vi "Dashboard Main.vi"() -> ()   [LabVIEW 2017]
uses:
  <vilib>/Utility/miscctls.llb/LVRowAndColumnTypeDef.ctl
  <vilib>/event_ctls.llb/eventvkey.ctl
  <vilib>/Rock Robotics/Network Tables/NT Read Numeric Array.vi
  <vilib>/Rock Robotics/WPI/Dashboard/WPI_DashboardLogging Global.vi
panel:
  in  "Camera Settings Right":T1={"Frame Rate"=30, "Compression"=30, "Size"=1, "DB Camera Config"=FALSE} {"Frame Rate" scale=1.0..30.0; "Compression" scale=100.0..-1.0; "Size" items=["640x480", "320x240", "160x120"]}
  in  "Camera Name Right":string(combo)="No Camera Selection"
  out "Camera Info":cluster{"Mbps LED":bool, "Mbps":dbl, "fps":dbl} {"fps" format="%#.1g"; "Mbps" format="%#.1g"}
  in  "Camera Settings":T1={"Frame Rate"=30, "Compression"=30, "Size"=1, "DB Camera Config"=FALSE} {"Frame Rate" scale=1.0..30.0; "Compression" scale=100.0..-1.0; "Size" items=["640x480", "320x240", "160x120"]}
  in  "TCP":refnum<k5>
  in  "Rec Mode":enum32{"Stop", "Record", "Playback"}(radio)
  out "Robot IP":string
  out "Image Message":string="Timeout in Camera Communications"
  in  "Dashboard Tab":T2(tab)
  in  "Select Robot Start Location":string(combo)="Select Robot Start Position ..."
  in  "String":string="Tom's Custom Dashboard 2018"
  in  "Select Auto":string(combo)="Select Autonomous ..."
  out "NT Connection":bool
  out "MotorChart R":cluster{"Numeric":dbl, "Numeric":dbl}(graph)
  out "MotorChart L":cluster{"Numeric":dbl, "Numeric":dbl}(graph)
  out "MotorSliders R":cluster{"MotorSlide1":dbl, "MotorSlide2":dbl} {"MotorSlide2" scale=-1.0..1.0 scale format="%#_2e"; "MotorSlide1" scale=-1.0..1.0 scale format="%#_2e"}
  out "MotorSliders L":cluster{"MotorSlide1":dbl, "MotorSlide2":dbl} {"MotorSlide2" scale=-1.0..1.0 scale format="%#_2e"; "MotorSlide1" scale=-1.0..1.0 scale format="%#_2e"}
  out "Gyro":dbl(knob) scale=0.0..360.0
  out "JS1 Z":dbl(slide) scale=-1.0..1.0 scale format="%#_2e"
  out "JS1 Graph":cluster{"X":dbl, "Y":dbl}[](graph)
  out "JS1 Buttons":T3
  out "JS2 Z":dbl(slide) scale=-1.0..1.0 scale format="%#_2e"
  out "JS2 Graph":cluster{"X":dbl, "Y":dbl}[](graph)
  out "JS2 Buttons":T3
  out "Mode":T4(ring)=enum."Auto Disabled"
  out "Camera Image Right":T5(plugin-control)
  in  "DB/String 9":string
  in  "DB/String 8":string
  in  "DB/String 7":string
  in  "DB/String 6":string
  in  "DB/String 5":string
  in  "DB/String 4":string
  in  "DB/String 3":string
  in  "DB/String 2":string
  in  "DB/String 1":string
  in  "DB/String 0":string
  in  "DB/Slider 0":dbl(slide) scale=0.0..5.0
  in  "DB/Slider 1":dbl(slide) scale=0.0..5.0
  in  "DB/Slider 2":dbl(slide) scale=0.0..5.0
  in  "DB/Slider 3":dbl(slide) scale=0.0..5.0
  out "DB/LED 3":bool
  out "DB/LED 2":bool
  out "DB/LED 1":bool
  out "DB/LED 0":bool
  in  "DB/Button 3":bool
  in  "DB/Button 2":bool
  in  "DB/Button 1":bool
  in  "DB/Button 0":bool caption="New Name"
  in  "Test Slider":dbl(slide) scale=0.0..100.0 scale format="%#_3g"
  in  "On/Off":bool caption="Solenoid"
  in  "Test Name":u16(ring) items=["Select the test to run..."]
  in  "Test Tree":string(tree)
  in  "Motor":cluster{"Value":dbl, "Enable":bool} {"Value" scale=-1.0..1.0 scale format="%#_3g"}
  out "Progress":T6 {"Test Progress" scale=0.0..100.0}
  in  "Rev/Fwd":cluster{"Forward":bool, "Reverse":bool}
  in  "Test Ring":u16(ring) items=["Monochrome", "Color"]
  out "Cmd Status":string
  in  "Execute Command":bool
  in  "Command Params":string[][](table)
  in  "Command Selection":i32(listbox)
  in  "CheckList":i32(listbox)
  out "Tree":string(tree)
  out "Camera Image":T5(plugin-control)
  out "Background":bool
  in  "Camera Name":string(combo)="No Camera Selection"
  # "HW"
  # "HW"
  # "Joysticks"
  # "Drive Motors"
  # "Front"
  # "Right"
  # "Left"
  # "Back"
  # "This tab is a great place for autonomous settings and robot-specific values.\nPlace controls and indicators inside this tab and match name to\nDashboard Variables on robot. You can also delete this comment."
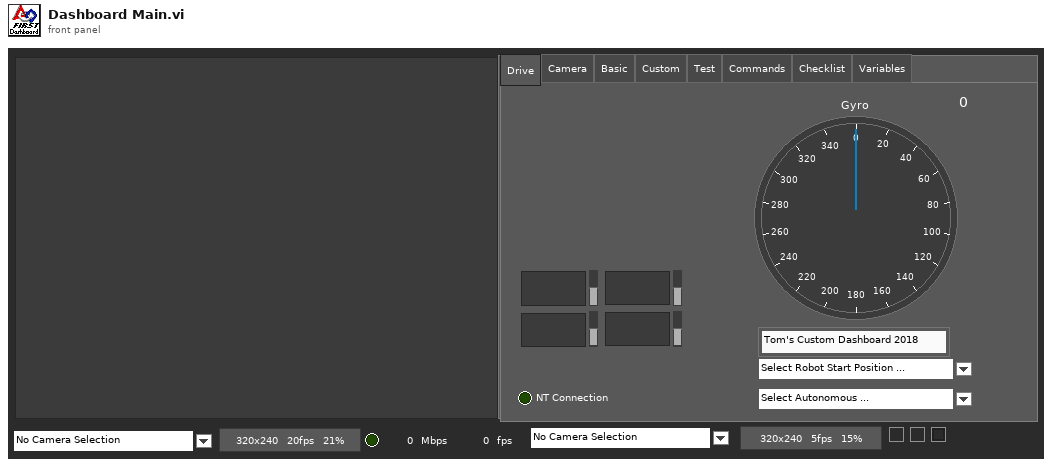
[diagram p1: front panel]
types:
  T1 = cluster{"Frame Rate":i32, "Compression":i32, "Size":u16, "DB Camera Config":bool}
  T2 = enum32{"Drive", "Camera", "Basic", "Custom", "Test", "Commands", "Checklist", "Variables"}
  T3 = cluster{bool, bool, bool, bool, bool, bool, bool, bool, bool, bool, bool, bool}
  T4 = enum8{"Tele-Op Disabled", "Tele-Op Enabled", "Auto Disabled", "Auto Enabled", "Test Disabled", "Test Enabled", "Disconnected", "No Code", "E-Stop"}
  T5 = typedef "IMAQ Image.ctl" = refnum<image>
  T6 = cluster{"Test Progress":u8, "Test Progress Text":string}
  T7 = cluster{"Save Path":path, "Interval (s)":dbl, "Keep":i32}
  T8 = typedef "Image Type" = u32
  T9 = cluster{"IDs":cluster{"RPC field ID":u16, "Unique ID":u16}, "String":string}
  T10 = cluster{"Error Strings":string, "Disable Counts":cluster{u16, u16}, "Rail Faults":cluster{u16, u16, u16}, "Robot IP":string, "DB Mode":u8, "Event Info":cluster{"Name":string, "Type":u8, "Number":u16, "Replay":u8}}
  T11 = cluster{"Storage":cluster{"Disk Free":u64, "RAM Block":u32, "RAM free":u32}, "CPU Utilization":cluster{"CPU % ISR":sgl, "CPU % Time Crit":sgl, "CPU % Timed Str":sgl, "CPU % High":sgl, "CPU % Above":sgl, "CPU % Normal":sgl, "CPU % Low":sgl}, "CAN":cluster{"% Bus Utilization":sgl, "Bus Off Cnt":u32, "TX_FIFO Full Cnt":u32, "Receive Error Cnt":u8, "Transmit Error Cnt":u8}, "HID":cluster{"HID Outputs":u32, "Rumble Low":u16, "Rumble High":u16}[]}
  T12 = cluster{"Status bits":cluster{"Test Mode":bool, "Autonomous":bool, "Enabled":bool, "Code Start":bool, "Brownout":bool, "Reserved 2":bool, "Reserved 3":bool, "E-Stop":bool}, "Code Trace":cluster{"Disabled":bool, "TeleOp":bool, "Auto":bool, "Test":bool}, "Controller Type":enum16{"unknown", "cRIO", "roboRio"}, "Code?":enum16{"unknown", "noCode", "code"}, "Battery V":dbl}
  T13 = cluster{"Control Bits":cluster{"TestMode":bool, "Autonomous":bool, "Enabled":bool, "FMS Present":bool, bool, bool, bool, "E-Stop":bool}, "Team Station ":u8, "Countdown":sgl, "Joystick Values":cluster{"Axes":dbl[], "Buttons":bool[], "POVs":i16[]}[]}
  T14 = cluster{"Axes":dbl[], "Buttons":bool[], "POVs":i16[]}[]
  T15 = cluster{"Axes":dbl[], "Buttons":bool[], "POVs":i16[]}
  T16 = cluster{"Buttons[0]":bool, "Buttons[1]":bool, "Buttons[2]":bool, "Buttons[3]":bool, "Buttons[4]":bool, "Buttons[5]":bool, "Buttons[6]":bool, "Buttons[7]":bool, "Buttons[8]":bool, "Buttons[9]":bool, "Buttons[10]":bool, "Buttons[11]":bool}
  T17 = cluster{"Camera Image":refnum<vi>, "Dashboard Tab":refnum<vi>, "Background":refnum<vi>, "Rec Mode":refnum<vi>, "Test Slider":refnum<vi>, "On/Off ":refnum<vi>, "Test Ring":refnum<vi>, "Rev/Fwd":refnum<vi>, "Test Name":refnum<vi>, "Motor":refnum<vi>, "Progress":refnum<vi>, "CheckList":refnum<vi>, "Tree":refnum<vi>, "Test Tree":refnum<vi>, "Command Params":refnum<vi>, "Command Selection":refnum<vi>, "Execute Command":refnum<vi>, "Cmd Status":refnum<vi>, "Camera Settings":refnum<vi>, "Camera Name":refnum<vi>, "Camera Info":refnum<vi>, "Camera Settings Right":refnum<vi>, "Camera Name Right":refnum<vi>, "Camera Image Right":refnum<vi>}
  T18 = cluster{"Camera Name":string, string, "Saved DB Images Info":cluster{"Save Path":path, "Interval (s)":dbl, "Keep":i32}}
  T19 = cluster{"Camera Name Right":string, string, "Saved DB Images Info":cluster{"Save Path":path, "Interval (s)":dbl, "Keep":i32}}
  T20 = cluster{"Operation":enum16{"Update", "Clear"}, "Color Box":u32}[]
  T21 = typedef "eventvkey.ctl" = enum16{"ASCII", "Enter", "Return", "Shift", "Ctrl", "Alt", "Cmd", "Opt", "Caps", "NumLock", "Clear", "Break", "Up", "Down", "Left", "Right", "Insert", "Delete", "Home", "End", "PageUp", "PageDown", "Escape", "Help", "Pause", "ScrollLock", "F1", "F2", "F3", "F4", "F5", "F6", "F7", "F8", "F9", "F10", "F11", "F12", "F13", "F14", "F15", "F16", "F17", "F18", "F19", "F20", "F21", "F22", "F23", "F24", "Play", "VolumeUp", "VolumeDown", "Mute", "Two Byte Char"}
  T22 = cluster{"Image Size":bool, "Image Type":bool, "Pixel Value":bool, "ROI Information":bool, "Zoom Factor":bool}
  T23 = cluster{"Operation":enum16{"Update", "Clear"}, "Color Box":u32}
  T24 = typedef "LVRowAndColumnTypeDef.ctl" = cluster{"Row":i32, "Column":i32}
  T25 = cluster{"Shift":bool, "Ctrl":bool, "Alt":bool, "Cmd":bool, "Opt":bool}
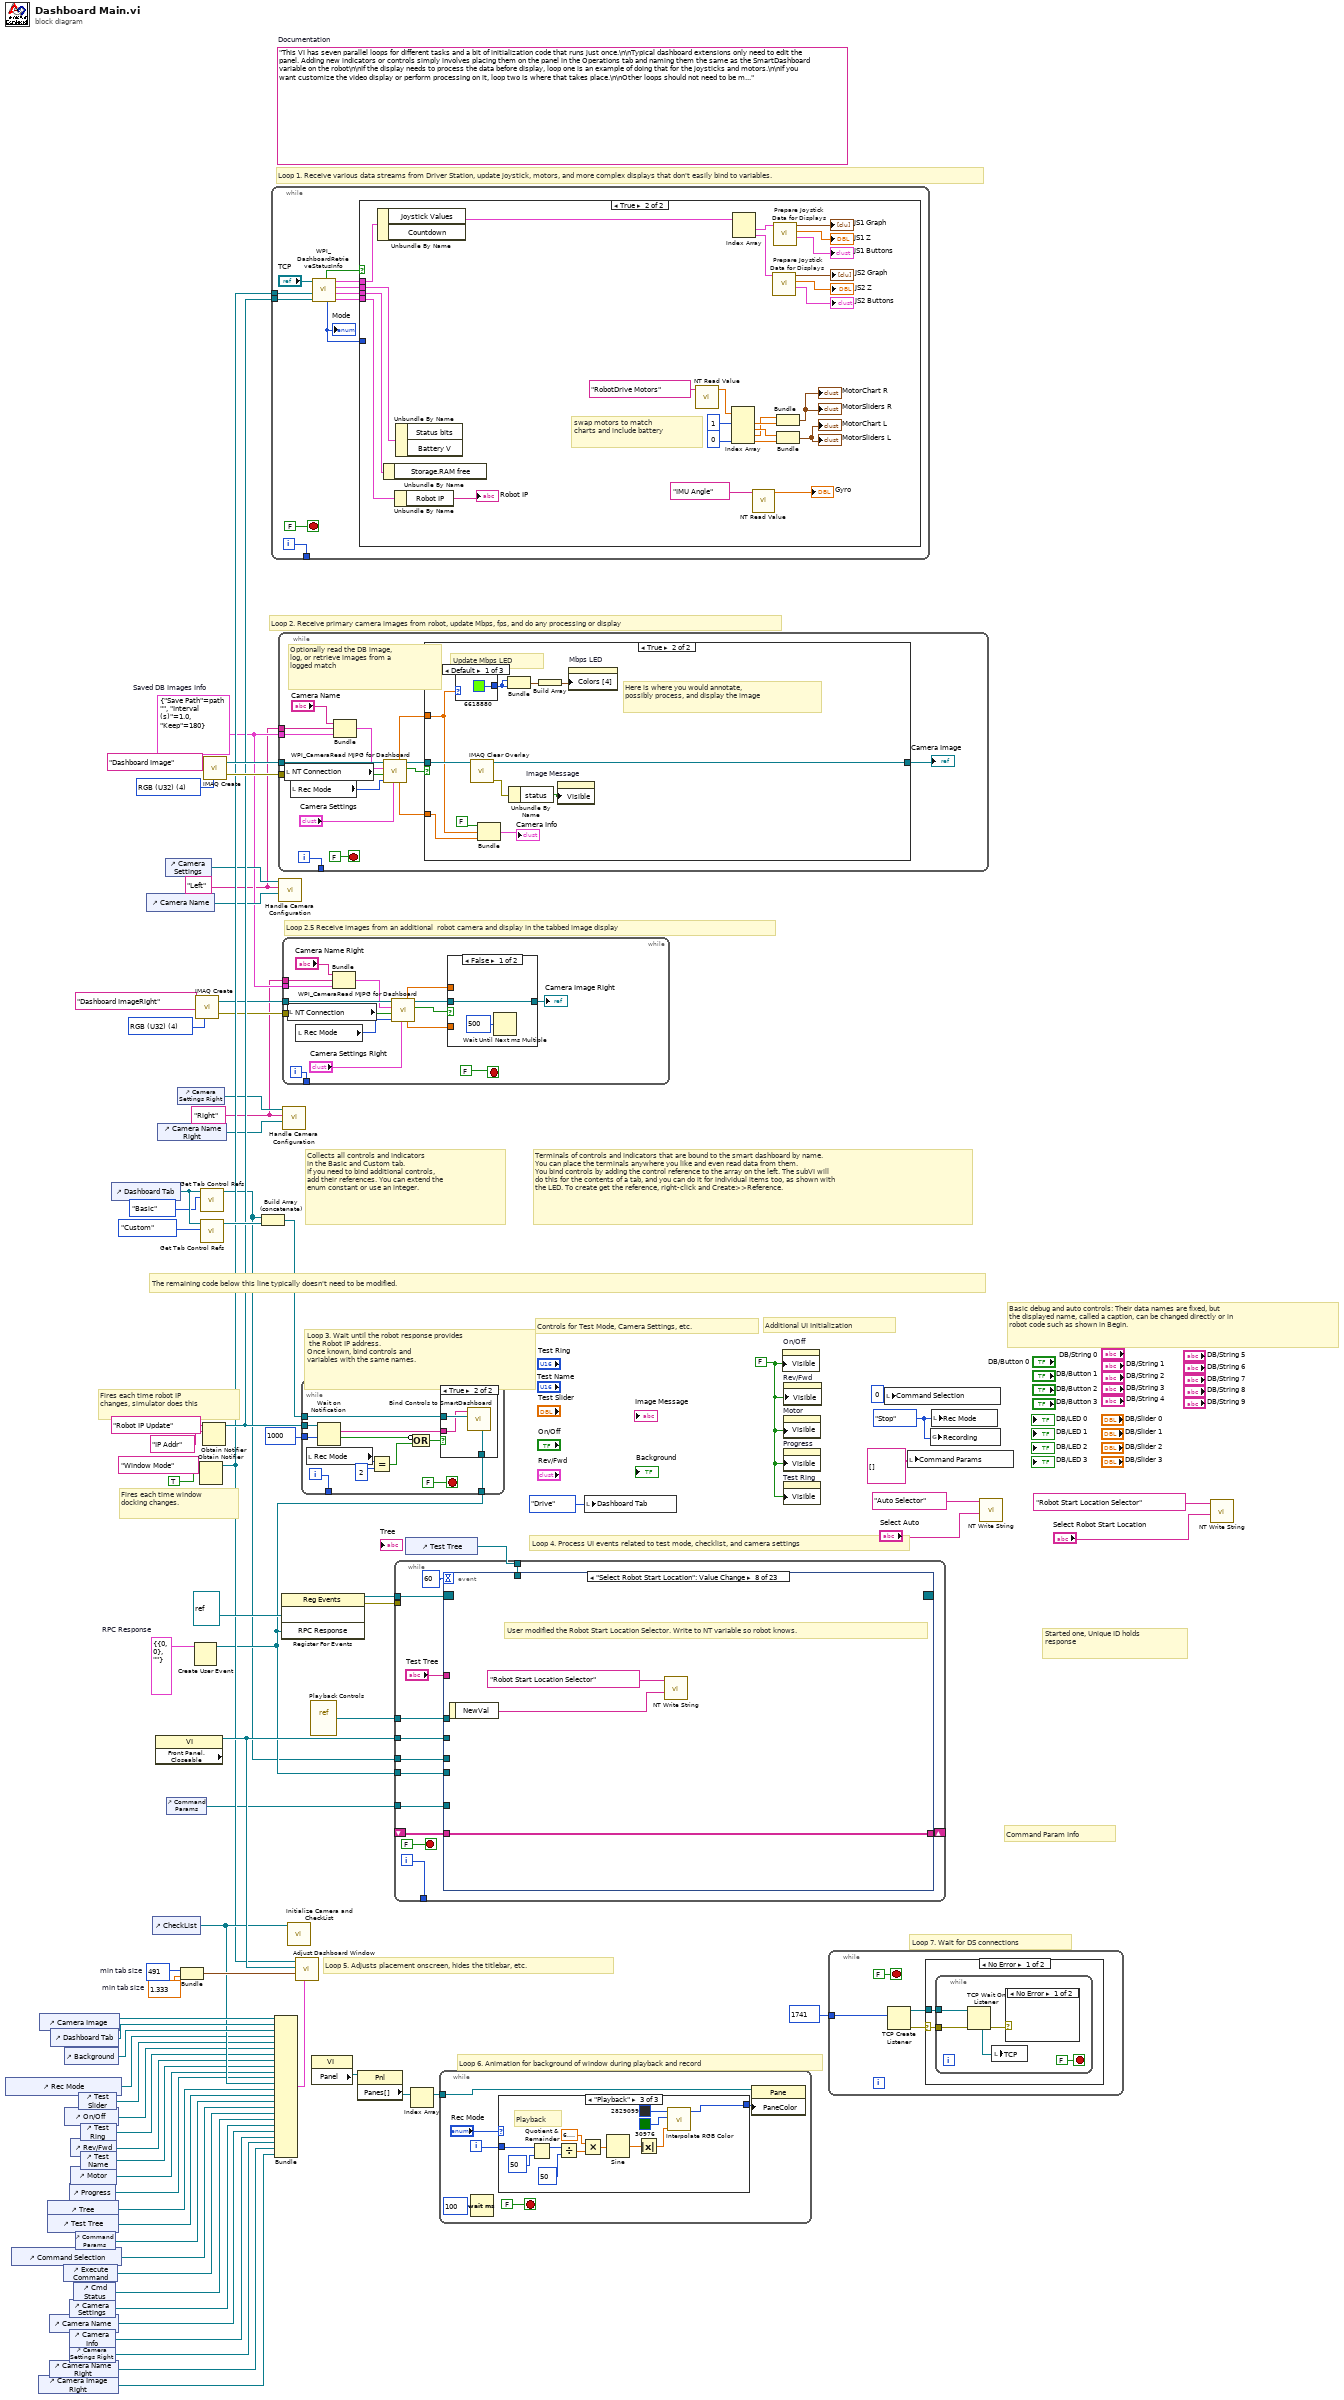
[diagram p0: block diagram]
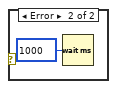
[diagram p3: hidden frame]
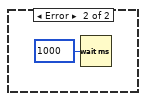
[diagram p4: hidden frame]
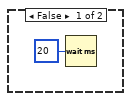
[diagram p5: hidden frame]
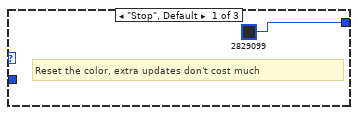
[diagram p6: hidden frame]
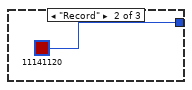
[diagram p7: hidden frame]
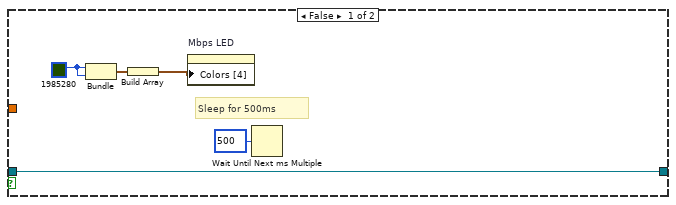
[diagram p9: hidden frame]
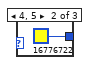
[diagram p10: hidden frame]
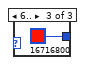
[diagram p11: hidden frame]
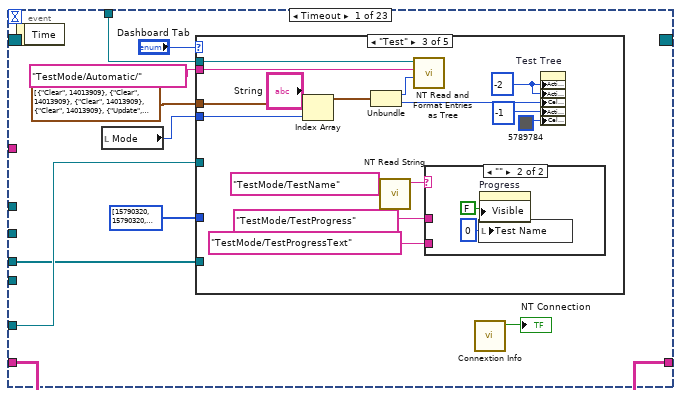
[diagram p12: hidden frame]
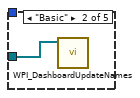
[diagram p14: hidden frame]
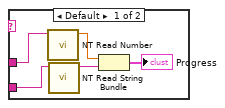
[diagram p15: hidden frame]
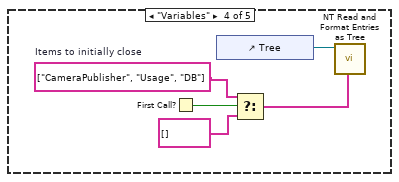
[diagram p16: hidden frame]
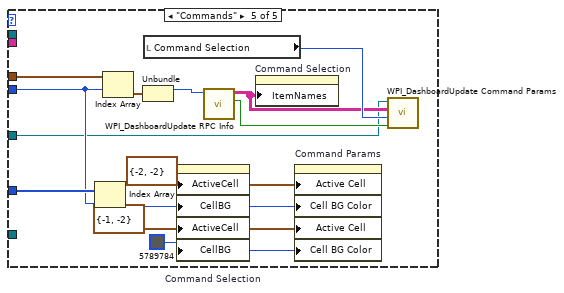
[diagram p17: hidden frame]
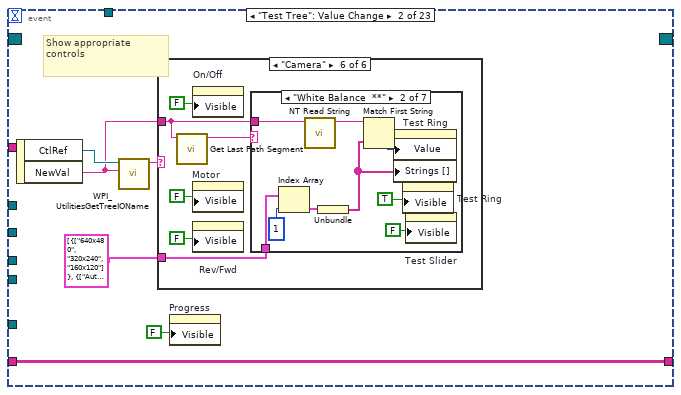
[diagram p18: hidden frame]
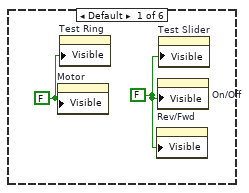
[diagram p19: hidden frame]
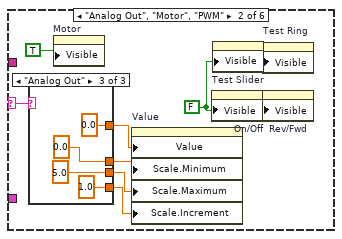
[diagram p20: hidden frame]
diagram:
  w5 = T7 {"Save Path"=path "", "Interval (s)"=1.0, "Keep"=180}  # Saved DB Images Info
  w4 = "Right"
  w3 = "Left"
  w15 = T8 4 items=["Grayscale (U8)", "Grayscale (I16)", "Grayscale (SGL)", "Complex (CSG)", "RGB (U32)", "HSL (U32)", "RGB (U64)"] ("Image Type")
  w31 = T9 {"IDs"={"RPC field ID"=0, "Unique ID"=0}, "String"=""}  # RPC Response
  w54 = 491  # min tab size
  w53 = 1.333  # min tab size
  w61 = enum32{"Stop", "Record", "Playback"}."Stop" ("Rec Mode")
  w38 = FALSE ("Visible")
  (unwired) "This VI has seven parallel loops for different tasks and a bit of initialization code that runs just once.\n\nTypical dashboard extensions only need to edit the panel. Adding new indicators or controls simply involves placing them on the panel in the Operations tab and naming them the same as the SmartDashboard variable on the robot\n\nIf the display needs to process the data before display, loop one is an example of doing that for the joysticks and motors.\n\nIf you want customize the video display or perform processing on it, loop two is where that takes place.\n\nOther loops should not need to be modified. They are pretty standard, and document the task they perform."  # Documentation
  w78 = T8 4 items=["Grayscale (U8)", "Grayscale (I16)", "Grayscale (SGL)", "Complex (CSG)", "RGB (U32)", "HSL (U32)", "RGB (U64)"] ("Image Type")
  # "Loop 2.5 Receive images from an additional  robot camera and display in the tabbed image display"
  # "Command Param Info"
  # "Started one, Unique ID holds\nresponse"
  # "Loop 7. Wait for DS connections"
  # "Basic debug and auto controls: Their data names are fixed, but\nthe displayed name, called a caption, can be changed directly or in\nrobot code such as shown in Begin."
  # "Controls for Test Mode, Camera Settings, etc."
  # "Additional UI Initialization"
  # "Loop 6. Animation for background of window during playback and record"
  # "Fires each time robot IP\nchanges, simulator does this"
  # "Fires each time window\ndocking changes."
  # "Collects all controls and indicators\nin the Basic and Custom tab.\nIf you need to bind additional controls,\nadd their references. You can extend the\nenum constant or use an integer."
  # "The remaining code below this line typically doesn't need to be modified."
  # "Loop 4. Process UI events related to test mode, checklist, and camera settings"
  # "Terminals of controls and indicators that are bound to the smart dashboard by name.\nYou can place the terminals anywhere you like and even read data from them.\nYou bind controls by adding the control reference to the array on the left. The subVI will\ndo this for the contents of a tab, and you can do it for individual items too, as shown with\nthe LED. To create get the reference, right-click and Create>>Reference."
  # "Loop 3. Wait until the robot response provides\n the Robot IP address.\nOnce known, bind controls and\nvariables with the same names."
  # "Loop 5. Adjusts placement onscreen, hides the titlebar, etc."
  # "Loop 1. Receive various data streams from Driver Station, update joystick, motors, and more complex displays that don't easily bind to variables."
  # "Loop 2. Receive primary camera images from robot, update Mbps, fps, and do any processing or display"
  n1 = control-ref of="Rec Mode"() -> (w44:refnum<vi>)
  n2 = control-ref of="Command Selection"() -> (w30:refnum<vi>)
  n3 = control-ref of="Camera Image Right"() -> (w8:refnum<vi>)
  n4 = control-ref of="Camera Image"() -> (w56:refnum<vi>)
  n5 = control-ref of="Tree"() -> (w48:refnum<vi>)
  n6 = control-ref of="Test Tree"() -> (w47:refnum<vi>)
  n7 = control-ref of="Camera Name"() -> (w21:refnum<vi>)
  n8 = control-ref of="Camera Name Right"() -> (w9:refnum<vi>)
  n9 = control-ref of="Dashboard Tab"() -> (w55:refnum<vi>)
  n10 = control-ref of="Execute Command"() -> (w32:refnum<vi>)
  n11 = control-ref of="Background"() -> (w51:refnum<vi>)
  n12 = control-ref of="On/Off"() -> (w42:refnum<vi>)
  n13 = control-ref of="Progress"() -> (w39:refnum<vi>)
  n14 = control-ref of="Camera Settings"() -> (w22:refnum<vi>)
  n15 = control-ref of="Camera Info"() -> (w20:refnum<vi>)
  n16 = control-ref of="Camera Settings Right"() -> (w10:refnum<vi>)
  n17 = control-ref of="Rev/Fwd"() -> (w40:refnum<vi>)
  n18 = control-ref of="Motor"() -> (w45:refnum<vi>)
  n19 = control-ref of="Cmd Status"() -> (w26:refnum<vi>)
  n20 = control-ref of="Command Params"() -> (w33:refnum<vi>)
  n21 = control-ref of="Test Slider"() -> (w43:refnum<vi>)
  n22 = control-ref of="Test Ring"() -> (w41:refnum<vi>)
  n23 = control-ref of="Test Name"() -> (w46:refnum<vi>)
  n24 = control-ref of="Dashboard Tab"() -> (w59:refnum<vi>)
  n25 = control-ref of="Camera Name"() -> (w23:refnum<vi>)
  n26 = control-ref of="CheckList"() -> (w49:refnum<vi>)
  n27 = property class="VI" props=["Front Panel.Closeable"]() -> (reference out=w60:refnum<vi>)  [unwired: 2 in, 2 out]
  n28 = control-ref of="Camera Name Right"() -> (w11:refnum<vi>)
  n29 = control-ref of="Camera Settings"() -> (w24:refnum<vi>)
  n30 = control-ref of="Command Params"() -> (w25:refnum<vi>)
  n31 = control-ref of="Camera Settings Right"() -> (w12:refnum<vi>)
  n32 = Bundle("min tab size"=w54, "min tab size"=w53) -> (w52:cluster{"min tab size":i32, "min tab size":dbl})  [unwired: 1 in]
  n33 = Create User Event(user event datatype=w31) -> (user event=w27:refnum<user-event>)  [unwired: 1 in, 1 out]
  n34 = call "IMAQ Create"("Image Name"="Dashboard ImageRight", "Image Type"=w15) -> ("New Image"=w14:T5, "error out"=w13:errorcluster)  [unwired: 2 in, 1 out]
  n35 = Obtain Notifier(name (unnamed)="Window Mode", notification data type=TRUE) -> (notifier out=w36:refnum<notifier>)  [unwired: 2 in, 2 out]
  n36 = call <vilib>:"Get Tab Control Refs.vi"("Page Index"=T2."Basic" ("Dashboard Tab"), "TabControl in"=w59) -> ("ControlsOnPage"=w19:refnum<vi>[])  [unwired: 9 in]
  n37 = call <vilib>:"Get Tab Control Refs.vi"("Page Index"=T2."Custom" ("Dashboard Tab"), "TabControl in"=w59) -> ("ControlsOnPage"=w58:refnum<vi>[])  [unwired: 9 in]
  n38 = Obtain Notifier(name (unnamed)="Robot IP Update", notification data type="IP Addr" ("name (unnamed)")) -> (notifier out=w37:refnum<notifier>)  [unwired: 2 in, 2 out]
  n39 = call "IMAQ Create"("Image Name"="Dashboard Image", "Image Type"=w78) -> ("New Image"=w76:T5, "error out"=w75:errorcluster)  [unwired: 2 in, 1 out]
  n40 = Build Array (concatenate)(w19, w58) -> (w57:refnum<vi>[])
  n41 = while {
    tunnel: [w88] -> _
    tunnel: w37 -> [w82]
    tunnel: w36 -> [w79]
    i -> [w88]
    stop <- FALSE stop-if-true
    n42 = call <vilib>:"WPI_DashboardRetrieveStatusInfo.vi"("Binding Refnum"=w82, "Window Mode Notifier"=w79, "TCP Cnx"="TCP") -> ("Power and Errors"=w83:T10, "Robot Metrics"=w86:T11, "Status Info"=w87:T12, "Control Info"=w84:T13, "Robot Mode"=w81:T4, "Process?"=w85:bool)  [unwired: 3 in]
    "Mode" <- w81
    n43 = case shown="True" w85 {
      tunnel: w87 -> [_ w116]
      tunnel: w86 -> [_ w115]
      tunnel: w84 -> [_ w114]
      tunnel: w83 -> [_ w113]
      tunnel: w81 -> [_ _]
      frame False {
        n44 = Wait (ms)(milliseconds to wait=u32 20) -> ()  [unwired: 1 out]
      }
      frame True {
        # "swap motors to match\ncharts and include battery"
        n45 = Unbundle By Name(w114) -> ("Joystick Values"=w104:T14)  [unwired: 1 out]
        n46 = Unbundle By Name(w115) -> ()  [unwired: 1 out]
        n47 = Unbundle By Name(w113) -> ("Robot IP"=→"Robot IP":string)
        n48 = Unbundle By Name(w116) -> ()  [unwired: 2 out]
        n49 = call-poly <vilib>:"NT Read Value.vi"("Name"="RobotDrive Motors") -> ("Numeric Array"=w94:dbl[])  [unwired: 9 in, 1 out]
        n50 = Index Array(array=w94, index #1=1, index #4=0) -> (element #1=w108:dbl, element #2=w109:dbl, element #3=w107:dbl, element #4=w112:dbl)  [unwired: 2 in]
        n51 = Index Array(array=w104) -> (element #1=w103:T15, element #2=w99:T15)  [unwired: 2 in]
        n52 = call-poly <vilib>:"NT Read Value.vi"("Name"="IMU Angle") -> ("Numeric"=→"Gyro":dbl)  [unwired: 9 in, 1 out]
        n53 = call "Prepare Joystick Data for Displays.vi"("Joystick Values"=w99) -> ("Buttons"=→"JS2 Buttons":T16, "Z Axis"=→"JS2 Z":dbl, "Cartesian Data"=→"JS2 Graph":cluster{"X axis":dbl, "X axis":dbl}[])  [unwired: 8 in]
        n54 = call "Prepare Joystick Data for Displays.vi"("Joystick Values"=w103) -> ("Buttons"=→"JS1 Buttons":T16, "Z Axis"=→"JS1 Z":dbl, "Cartesian Data"=→"JS1 Graph":cluster{"X axis":dbl, "X axis":dbl}[])  [unwired: 8 in]
        n55 = Bundle("Numeric"=w107, "Numeric"=w108) -> (→"MotorChart R" →"MotorSliders R":cluster{"Numeric":dbl, "Numeric":dbl})  [unwired: 1 in]
        n56 = Bundle("Numeric"=w109, "Numeric"=w112) -> (→"MotorChart L" →"MotorSliders L":cluster{"Numeric":dbl, "Numeric":dbl})  [unwired: 1 in]
      }
    }
  }
  n57 = Bundle("Camera Image"=w56, "Dashboard Tab"=w55, "Background"=w51, "Rec Mode"=w44, "Test Slider"=w43, "On/Off"=w42, "Test Ring"=w41, "Rev/Fwd"=w40, "Test Name"=w46, "Motor"=w45, "Progress"=w39, "CheckList"=w49, "Tree"=w48, "Test Tree"=w47, "Command Params"=w33, "Command Selection"=w30, "Execute Command"=w32, "Cmd Status"=w26, "Camera Settings"=w22, "Camera Name"=w21, "Camera Info"=w20, "Camera Settings Right"=w10, "Camera Name Right"=w9, "Camera Image Right"=w8) -> (w50:T17)  [unwired: 1 in]
  n58 = call "Handle Camera Configuration.vi"("CameraNameRef"=w23, "Display Name"=w3, "ClusterRef"=w24) -> ()  [unwired: 9 in]
  n59 = while {
    tunnel: w76 -> [w129]
    tunnel: w75 -> [_]
    tunnel: [w130] -> _
    tunnel: w5 -> [w120]
    tunnel: w3 -> [w117]
    i -> [w130]
    stop <- FALSE stop-if-true
    # "Optionally read the DB image,\nlog, or retrieve images from a\nlogged match"
    n60 = local read "NT Connection"() -> (w121:bool)
    n61 = local read "Rec Mode"() -> (w125:enum32{"Stop", "Record", "Playback"})
    n62 = Bundle("Camera Name"="Camera Name", w117, "Saved DB Images Info"=w120) -> (w119:T18)  [unwired: 1 in]
    n63 = call <vilib>:"WPI_CameraRead MJPG for Dashboard.vi"("Camera Settings"="Camera Settings", "Rec Mode"=w125, "NT Connection"=w121, "Capture Info"=w119, "Refnum in"=w129) -> ("Active"=w127:bool, "Refnum out"=w128:T5, "FPS"=w126:dbl, "Bandwidth (Mbps)"=w124:dbl)  [unwired: 3 in]
    n64 = case shown="True" w127 {
      tunnel: w128 -> [w132 w143]
      tunnel: w124 -> [_ w140]
      tunnel: w126 -> [_ w141]
      tunnel: [w132 w137] -> w122
      frame False {
        w134 = u32 1985280 ("Color Box")
        # "Sleep for 500ms"
        n65 = Bundle("Color Box"=w134, "Color Box"=w134) -> (w135:cluster{"Color Box":u32, "Color Box":u32})  [unwired: 1 out]
        n66 = Build Array(w135) -> (w133:cluster{"Color Box":u32, "Color Box":u32}[])
        n67 = property on="Mbps LED" class="Bool (strict)"("Colors [4]"=w133) -> ()  [unwired: 2 in, 2 out]
        n68 = Wait Until Next ms Multiple(millisecond multiple=u32 500) -> ()  [unwired: 1 out]
      }
      frame True {
        # "Here is where you would annotate,\npossibly process, and display the image"
        # "Update Mbps LED"
        n69 = case shown="Default" w140 {
          tunnel: [u32 6618880 ("Color Box") u32 16776722 ("Color Box") u32 16716800 ("Color Box")] -> w144
          frame Default {
          }
          frame 4, 5 {
          }
          frame 6.. {
          }
        }
        n70 = call "IMAQ Clear Overlay"("Image"=w143) -> ("error out"=w146:errorcluster, "Image Out"=w137:T5)  [unwired: 2 in, 7 out]
        n71 = Bundle(FALSE, "Bandwidth (Mbps)"=w140, "FPS"=w141) -> (→"Camera Info":cluster{bool, "Bandwidth (Mbps)":dbl, "FPS":dbl})  [unwired: 1 in]
        n72 = Bundle("Color Box"=w144, "Color Box"=w144) -> (w145:cluster{"Color Box":u32, "Color Box":u32})  [unwired: 1 out]
        n73 = Unbundle By Name(w146) -> ("status"=w147:bool)
        n74 = Build Array(w145) -> (w142:cluster{"Color Box":u32, "Color Box":u32}[])
        n75 = property on="Image Message" class="Str"("Visible"=w147) -> ()  [unwired: 2 in, 2 out]
        n76 = property on="Mbps LED" class="Bool (strict)"("Colors [4]"=w142) -> ()  [unwired: 2 in, 2 out]
      }
    }
    "Camera Image" <- w122
  }
  n77 = register-events(refnum<vi> refnum, w27) -> (reference out=w65:refnum<event-registration>, error out=w64:errorcluster)  [unwired: 2 in]
  n78 = while {
    tunnel: w14 -> [w165]
    tunnel: w13 -> [_]
    tunnel: [w160] -> _
    tunnel: w5 -> [w154]
    tunnel: w4 -> [w151]
    i -> [w160]
    stop <- FALSE stop-if-true
    n79 = local read "NT Connection"() -> (w155:bool)
    n80 = local read "Rec Mode"() -> (w164:enum32{"Stop", "Record", "Playback"})
    n81 = Bundle("Camera Name Right"="Camera Name Right", w151, "Saved DB Images Info"=w154) -> (w153:T19)  [unwired: 1 in]
    n82 = call <vilib>:"WPI_CameraRead MJPG for Dashboard.vi"("Camera Settings"="Camera Settings Right", "Rec Mode"=w164, "NT Connection"=w155, "Capture Info"=w153, "Refnum in"=w165) -> ("Active"=w159:bool, "Refnum out"=w162:T5, "FPS"=w157:dbl, "Bandwidth (Mbps)"=w158:dbl)  [unwired: 3 in]
    n83 = case shown="False" w159 {
      tunnel: w162 -> [w166 w168]
      tunnel: w158 -> [_ _]
      tunnel: w157 -> [_ _]
      tunnel: [w166 w168] -> w156
      frame False {
        n84 = Wait Until Next ms Multiple(millisecond multiple=u32 500) -> ()  [unwired: 1 out]
      }
      frame True {
      }
    }
    "Camera Image Right" <- w156
  }
  n85 = call "Handle Camera Configuration.vi"("CameraNameRef"=w11, "Display Name"=w4, "ClusterRef"=w12) -> ()  [unwired: 9 in]
  n86 = call "Initialize Camera and CheckList.vi"("ListBox in"=w49) -> ()  [unwired: 11 in]
  n87 = call "Adjust Dashboard Window.vi"("Sizing Refnums"=w50, "Size Constraints"=w52, "VI"=w60, "WIn Mode"=w36) -> ()  [unwired: 8 in]
  n88 = while {
    tunnel: w57 -> [w180]
    tunnel: w37 -> [w178]
    tunnel: [w176] -> _
    tunnel: u32 1000 ("milliseconds to wait") -> [w175]
    tunnel: w27 -> [w169]
    i -> [w176]
    stop <- FALSE stop-if-true
    n89 = local read "Rec Mode"() -> (w171:enum32{"Stop", "Record", "Playback"})
    n90 = Wait on Notification(notifier=w178, timeout in ms (-1)=w175) -> (notification=w177:string, timed out?=w173:bool)  [unwired: 2 in, 2 out]
    n91 = Equal?(x=w171, y=u16 2 ("Rec Mode")) -> (x = y?=w172:bool)
    n92 = Compound Arithmetic op=OR(invert w173, w172) -> (w174:bool)
    n93 = case shown="True" w174 {
      tunnel: w180 -> [_ w183]
      tunnel: w177 -> [_ w182]
      tunnel: w169 -> [_ w181]
      frame False {
      }
      frame True {
        n94 = call <vilib>:"Bind Controls to SmartDashboard.vi"("RPC ref"=w181, "Bound Control Refs"=w183, "Server IP Address"=w182) -> ()  [unwired: 9 in]
      }
    }
  }
  n95 = vi-ref "Playback Controls.vi"() -> (w66:refnum<vi>)
  n96 = property class="VI"() -> ("Panel"=w68:refnum<vi>)  [unwired: 2 in, 2 out]
  n97 = property class="Pnl"(reference=w68) -> ("Panes[]"=w69:refnum<vi>[])  [unwired: 1 in, 2 out]
  n98 = control-ref of="Test Tree"() -> (w70:refnum<vi>)
  n99 = while {
    tunnel: [w193] -> _
    tunnel: w70 -> [w192]
    tunnel: w66 -> [w191]
    tunnel: w65 -> [w190]
    tunnel: w64 -> [_]
    tunnel: w60 -> [w189]
    tunnel: w27 -> [w188]
    tunnel: w25 -> [w187]
    shift-right: [w186] -> _
    shift-left: _ -> [w185]
    tunnel: w19 -> [w184]
    i -> [w193]
    stop <- FALSE stop-if-true
    n100 = event shown="[7] \"Select Robot Start Location\": Value Change" {
      selector: w190 -> [_ _ _ _ _ _ _ _ _ _ _ _ _ _ _ _ _ _ _ _ _ _ _]
      dyn-events: [_ _ _ _ _ _ _ _ _ _ _ _ _ _ _ _ _ _ w459 _ _ _ _] -> _
      timeout: u32 60 ("milliseconds to wait") -> [_ _ _ _ _ _ _ _ _ _ _ _ _ _ _ _ _ _ _ _ _ _ _]
      tunnel: w192 -> [w205 _ _ _ _ _ _ _ _ _ _ _ _ _ _ _ _ _ _ _ _ _ _]
      tunnel: "Test Tree" -> [_ _ _ _ _ _ _ _ _ _ _ _ _ w426 w434 w436 w440 w448 _ _ _ _ _]
      tunnel: w191 -> [_ _ _ _ _ _ _ _ _ _ _ _ _ _ _ _ _ _ w461 _ w479 _ _]
      tunnel: w189 -> [_ _ _ _ _ _ _ _ _ _ _ _ _ _ _ _ _ _ w457 _ _ _ _]
      tunnel: w188 -> [_ _ _ _ _ _ _ _ _ _ _ _ _ _ _ _ _ _ w455 _ _ _ _]
      tunnel: w187 -> [w200 _ _ _ _ _ _ _ w377 _ _ _ _ _ _ _ _ _ _ _ _ _ _]
      tunnel: [w199 w248 w350 w355 w364 w368 w371 w374 w375 w384 w394 w401 w413 w425 w432 w435 w439 w447 w454 w474 w476 w480 w493] -> w186
      tunnel: w185 -> [w199 w248 w350 w355 w364 w368 w371 w374 w375 _ _ w401 w413 w425 w432 w435 w439 w447 w454 w474 w476 w480 w493]
      tunnel: w184 -> [w197 _ _ _ _ _ _ _ _ _ _ _ _ _ _ _ _ _ _ _ _ _ _]
      event Timeout {
        n101 = event-data() -> ()  [unwired: 1 in, 1 out]
        n102 = local read "Mode"() -> (w202:T4)
        n103 = case shown="\"Test\"" "Dashboard Tab" {
          tunnel: w205 -> [_ _ w221 _ _]
          tunnel: "TestMode/Automatic/" ("Name Pattern") -> [_ _ w220 _ _]
          tunnel: T20 [{"Operation"=enum."Clear", "Color Box"=14013909}, {"Operation"=enum."Clear", "Color Box"=14013909}, {"Operation"=enum."Clear", "Color Box"=14013909}, {"Operation"=enum."Clear", "Color Box"=14013909}, {"Operation"=enum."Update", "Color Box"=14013909}, {"Operation"=enum."Update", "Color Box"=16777215}, {"Operation"=enum."Clear", "Color Box"=14013909}, {"Operation"=enum."Clear", "Color Box"=14013909}, {"Operation"=enum."Clear", "Color Box"=14013909}] -> [_ _ w213 _ w241]
          tunnel: w202 -> [_ _ w212 _ w240]
          tunnel: u32[] [15790320, 15790320, 15790320, 15790320, 16777215, 16777215, 15790320, 15790320, 15790320] -> [_ _ _ _ w246]
          tunnel: w200 -> [_ _ _ _ w234]
          tunnel: w197 -> [_ w207 _ _ _]
          frame "Custom", Default {
          }
          frame "Basic" {
            n104 = call <vilib>:"WPI_DashboardUpdateNames.vi"("Controls on Tab"=w207) -> ()  [unwired: 11 in]
          }
          frame "Test" {
            w219 = -2 ("Active Item:Row Number")
            n105 = Index Array(array=w213, index=w212) -> (element=w214:T23)
            n106 = Unbundle(w214) -> ("Operation"=w215:enum16{"Update", "Clear"}, "Color Box"=w216:u32)
            n107 = call <vilib>:"NT Read String.vi"("Name"="TestMode/TestName") -> ("String"=w210:string)  [unwired: 9 in, 1 out]
            n108 = call <vilib>:"NT Read and Format Entries as Tree.vi"("Operation"=w215, "Name Pattern"=w220, "Tree Refnum"=w221) -> ()  [unwired: 7 in, 2 out]
            n109 = case shown="\"\"" w210 {
              tunnel: "TestMode/TestProgress" ("Name") -> [w223 _]
              tunnel: "TestMode/TestProgressText" ("Name") -> [w222 _]
              frame Default {
                n110 = call <vilib>:"NT Read Number.vi"("Name"=w223) -> ("Numeric"=w224:dbl)  [unwired: 9 in, 1 out]
                n111 = call <vilib>:"NT Read String.vi"("Name"=w222) -> ("String"=w225:string)  [unwired: 9 in, 1 out]
                n112 = Bundle("Numeric"=w224, "String"=w225) -> (→"Progress":cluster{"Numeric":dbl, "String":string})  [unwired: 1 in]
              }
              frame "" {
                n113 = local write "Test Name"(u16 0) -> ()
                n114 = property on="Progress" class="Clust (strict)"("Visible"=FALSE) -> ()  [unwired: 2 in, 2 out]
              }
            }
            n115 = property on="Test Tree" class="Tree (strict)"("Active Item Row Number"=w219, "ActiveColNum"=w219, "CellBG"=w216, "Active Item Row Number"=-1 ("Active Item:Row Number"), "CellBG"=u32 5789784 ("Color Box")) -> ()  [unwired: 2 in, 2 out]
          }
          frame "Variables" {
            w231 = string[] ["CameraPublisher", "Usage", "DB"]  # Items to initially close
            n116 = First Call?() -> (First Call?: T/F=w232:bool)
            n117 = control-ref of="Tree"() -> (w233:refnum<vi>)
            n118 = Select(t=w231, s=w232, f=string[] []) -> (s? t:f=w229:string[])
            n119 = call <vilib>:"NT Read and Format Entries as Tree.vi"("Tags to  Close"=w229, "Tree Refnum"=w233) -> ()  [unwired: 8 in, 2 out]
          }
          frame "Commands" {
            w242 = u32 5789784 ("Color Box")
            w243 = T24 {"Row"=-1, "Column"=-2} ("Active Cell:Active Cell")
            w245 = T24 {"Row"=-2, "Column"=-2} ("Active Cell:Active Cell")
            n120 = Index Array(array=w246, index=w240) -> (element=w244:u32)
            n121 = Index Array(array=w241, index=w240) -> (element=w239:T23)
            n122 = Unbundle(w239) -> ("Operation"=w238:enum16{"Update", "Clear"})  [unwired: 1 out]
            n123 = local read "Command Selection"() -> (w237:i32)
            n124 = property on="Command Selection" class="MCListbox (strict)"("ActiveCell"=w245, "CellBG"=w244, "ActiveCell"=w243, "CellBG"=w242) -> ()  [unwired: 2 in, 2 out]
            n125 = call <vilib>:"WPI_DashboardUpdate RPC Info.vi"("Operation"=w238) -> ("update"=w236:bool, "commands"=w235:string[][])  [unwired: 9 in]
            n126 = property on="Command Selection" class="MCListbox (strict)"("ItemNames"=w235) -> ()  [unwired: 2 in, 2 out]
            n127 = property on="Command Params" class="Tbl (strict)"("Active Cell"=w245, "Cell BG Color"=w244, "Active Cell"=w243, "Cell BG Color"=w242) -> ()  [unwired: 2 in, 2 out]
            n128 = call <vilib>:"WPI_DashboardUpdate Command Params.vi"("Update"=w236, "NewVal"=w237, "Commands"=w235, "Param Tbl"=w234) -> ()  [unwired: 7 in, 1 out]
          }
        }
        n129 = call <vilib>:"Connextion Info.vi"() -> ("Connected"=→"NT Connection":bool)  [unwired: 10 in, 1 out]
      }
      event "Test Tree": Value Change {
        # "Show appropriate\ncontrols"
        n130 = event-data() -> ("CtlRef"=w251:refnum<vi>, "NewVal"=w249:string)  [unwired: 1 in]
        n131 = call <vilib>:"WPI_UtilitiesGetTreeIOName.vi"("NewVal"=w249, "TreeControl in"=w251) -> ("I/O Name"=w252:string)  [unwired: 9 in]
        n132 = case shown="\"Camera\"" w252 {
          selector: w252 -> [_ w259 _ w281 w290 _]
          tunnel: w249 -> [_ _ w278 w280 _ w297]
          tunnel: cluster{string[]}[] [{["640x480", "320x240", "160x120"]}, {["Auto", "Fixed indoor", "Fixed outdoor 1", "Fixed outdoor 2", "Fixed fluorescent 1", "Fixed fluorescent 2", "Hold current"]}, {["Auto", "Flicker-free 50 Hz", "Flicker-free 60 Hz", "Hold current"]}, {["None", "Prioritize frame rate", "Prioritize image quality"]}, {["Monochrome", "Color"]}] -> [_ _ _ _ _ w296]
          frame Default {
            w254 = FALSE ("Visible")
            w253 = FALSE ("Visible")
            n133 = property on="Motor" class="Clust (strict)"("Visible"=w253) -> ()  [unwired: 2 in, 2 out]
            n134 = property on="Test Ring" class="Ring (strict)"("Visible"=w253) -> ()  [unwired: 2 in, 2 out]
            n135 = property on="Rev/Fwd" class="Clust (strict)"("Visible"=w254) -> ()  [unwired: 2 in, 2 out]
            n136 = property on="On/Off" class="Bool (strict)"("Visible"=w254) -> ()  [unwired: 2 in, 2 out]
            n137 = property on="Test Slider" class="Slide (strict)"("Visible"=w254) -> ()  [unwired: 2 in, 2 out]
          }
          frame "Analog Out", "Motor", "PWM" {
            w260 = FALSE ("Visible")
            n138 = case shown="\"Analog Out\"" w259 {
              tunnel: [1.0 ("Value") -1.0 ("Value") 0.0 ("Value")] -> w258
              tunnel: [255.0 ("Value") 1.0 ("Value") 5.0 ("Value")] -> w257
              tunnel: [128.0 ("Value") 0.0 ("Value") 0.0 ("Value")] -> w256
              tunnel: [64.0 ("Value") 0.5 ("Value") 1.0 ("Value")] -> w255
              frame "PWM" {
              }
              frame "Motor", Default {
              }
              frame "Analog Out" {
              }
            }
            n139 = property on="Motor" class="Clust (strict)"("Visible"=TRUE) -> ()  [unwired: 2 in, 2 out]
            n140 = property on="Value" class="Slide (strict)"("Value"=w256, "Scale.Minimum"=w258, "Scale.Maximum"=w257, "Scale.Increment"=w255) -> ()  [unwired: 2 in, 2 out]
            n141 = property on="On/Off" class="Bool (strict)"("Visible"=w260) -> ()  [unwired: 2 in, 2 out]
            n142 = property on="Test Slider" class="Slide (strict)"("Visible"=w260) -> ()  [unwired: 2 in, 2 out]
            n143 = property on="Test Ring" class="Ring (strict)"("Visible"=w260) -> ()  [unwired: 2 in, 2 out]
            n144 = property on="Rev/Fwd" class="Clust (strict)"("Visible"=w260) -> ()  [unwired: 2 in, 2 out]
          }
          frame "Servo" {
            w276 = FALSE ("Visible")
            n145 = call <vilib>:"NT Read Number.vi"("Name"=w278) -> ("Numeric"=w277:dbl)  [unwired: 9 in, 1 out]
            n146 = property on="Test Slider" class="Slide (strict)"("Visible"=TRUE, "Scale.Maximum"=170.0 ("Scale.Range:Maximum")) -> ()  [unwired: 2 in, 2 out]
            n147 = local write "Test Slider"(w277) -> ()
            n148 = property on="Motor" class="Clust (strict)"("Visible"=w276) -> ()  [unwired: 2 in, 2 out]
            n149 = property on="Rev/Fwd" class="Clust (strict)"("Visible"=w276) -> ()  [unwired: 2 in, 2 out]
            n150 = property on="On/Off" class="Bool (strict)"("Visible"=w276) -> ()  [unwired: 2 in, 2 out]
            n151 = property on="Test Ring" class="Ring (strict)"("Visible"=w276) -> ()  [unwired: 2 in, 2 out]
          }
          frame "Relay", "Solenoid" {
            w279 = FALSE ("Visible")
            n152 = property on="Motor" class="Clust (strict)"("Visible"=w279) -> ()  [unwired: 2 in, 2 out]
            n153 = property on="Test Slider" class="Slide (strict)"("Visible"=w279) -> ()  [unwired: 2 in, 2 out]
            n154 = Search and Replace String(input string=w280, search string="/Value  **", replace string="/Direction") -> (result string=w286:string)  [unwired: 5 in, 3 out]
            n155 = property on="Test Ring" class="Ring (strict)"("Visible"=w279) -> ()  [unwired: 2 in, 2 out]
            n156 = call <vilib>:"NT Read String.vi"("Name"=w286) -> ("String"=w284:string)  [unwired: 9 in, 1 out]
            n157 = Equal?(x="Both directions", y=w284) -> (x = y?=w282:bool)
            n158 = Not(x=w282) -> (.not. x?=w283:bool)
            n159 = property on="Rev/Fwd" class="Clust (strict)"("Visible"=w282) -> ()  [unwired: 2 in, 2 out]
            n160 = property on="On/Off" class="Bool (strict)"("Visible"=w283, "Caption.Text"=w281) -> ()  [unwired: 2 in, 2 out]
          }
          frame "Compressor", "Digital Out" {
            w289 = FALSE ("Visible")
            # "Get direction and finish"
            n161 = property on="Motor" class="Clust (strict)"("Visible"=w289) -> ()  [unwired: 2 in, 2 out]
            n162 = property on="Test Slider" class="Slide (strict)"("Visible"=w289) -> ()  [unwired: 2 in, 2 out]
            n163 = property on="Test Ring" class="Ring (strict)"("Visible"=w289) -> ()  [unwired: 2 in, 2 out]
            n164 = property on="On/Off" class="Bool (strict)"("Visible"=TRUE, "Caption.Text"=w290) -> ()  [unwired: 2 in, 2 out]
            n165 = property on="Rev/Fwd" class="Clust (strict)"("Visible"=FALSE) -> ()  [unwired: 2 in, 2 out]
          }
          frame "Camera" {
            n166 = call <vilib>:"Get Last Path Segment.vi"("String in"=w297) -> ("String out"=w298:string)  [unwired: 10 in]
            n167 = property on="On/Off" class="Bool (strict)"("Visible"=FALSE) -> ()  [unwired: 2 in, 2 out]
            n168 = property on="Motor" class="Clust (strict)"("Visible"=FALSE) -> ()  [unwired: 2 in, 2 out]
            n169 = property on="Rev/Fwd" class="Clust (strict)"("Visible"=FALSE) -> ()  [unwired: 2 in, 2 out]
            n170 = case shown="\"White Balance  **\"" w298 {
              tunnel: w297 -> [w304 w313 w322 w331 w340 _ w346]
              tunnel: w296 -> [w302 w310 w319 w328 w337 _ _]
              frame "Size  **" {
                n171 = Index Array(array=w302) -> (element=w301:cluster{string[]})  [unwired: 1 in]
                n172 = call <vilib>:"NT Read String.vi"("Name"=w304) -> ("String"=w303:string)  [unwired: 9 in, 1 out]
                n173 = Unbundle(w301) -> (w299:string[])
                n174 = Match First String(2:w299, 3:w303) -> (0:w300:i32)  [unwired: 1 out]
                n175 = property on="Test Ring" class="Ring (strict)"("Value"=w300, "Strings []"=w299) -> ()  [unwired: 2 in, 2 out]
                n176 = property on="Test Ring" class="Ring (strict)"("Visible"=TRUE) -> ()  [unwired: 2 in, 2 out]
                n177 = property on="Test Slider" class="Slide (strict)"("Visible"=FALSE) -> ()  [unwired: 2 in, 2 out]
              }
              frame "White Balance  **" {
                n178 = Index Array(array=w310, index=1) -> (element=w311:cluster{string[]})
                n179 = call <vilib>:"NT Read String.vi"("Name"=w313) -> ("String"=w312:string)  [unwired: 9 in, 1 out]
                n180 = Unbundle(w311) -> (w308:string[])
                n181 = Match First String(2:w308, 3:w312) -> (0:w307:i32)  [unwired: 1 out]
                n182 = property on="Test Ring" class="Ring (strict)"("Value"=w307, "Strings []"=w308) -> ()  [unwired: 2 in, 2 out]
                n183 = property on="Test Ring" class="Ring (strict)"("Visible"=TRUE) -> ()  [unwired: 2 in, 2 out]
                n184 = property on="Test Slider" class="Slide (strict)"("Visible"=FALSE) -> ()  [unwired: 2 in, 2 out]
              }
              frame "Exposure  **" {
                n185 = Index Array(array=w319, index=2) -> (element=w320:cluster{string[]})
                n186 = call <vilib>:"NT Read String.vi"("Name"=w322) -> ("String"=w321:string)  [unwired: 9 in, 1 out]
                n187 = Unbundle(w320) -> (w316:string[])
                n188 = Match First String(2:w316, 3:w321) -> (0:w317:i32)  [unwired: 1 out]
                n189 = property on="Test Ring" class="Ring (strict)"("Value"=w317, "Strings []"=w316) -> ()  [unwired: 2 in, 2 out]
                n190 = property on="Test Ring" class="Ring (strict)"("Visible"=TRUE) -> ()  [unwired: 2 in, 2 out]
                n191 = property on="Test Slider" class="Slide (strict)"("Visible"=FALSE) -> ()  [unwired: 2 in, 2 out]
              }
              frame "Exposure Priority  **" {
                n192 = Index Array(array=w328, index=3) -> (element=w329:cluster{string[]})
                n193 = call <vilib>:"NT Read String.vi"("Name"=w331) -> ("String"=w330:string)  [unwired: 9 in, 1 out]
                n194 = Unbundle(w329) -> (w325:string[])
                n195 = Match First String(2:w325, 3:w330) -> (0:w326:i32)  [unwired: 1 out]
                n196 = property on="Test Ring" class="Ring (strict)"("Value"=w326, "Strings []"=w325) -> ()  [unwired: 2 in, 2 out]
                n197 = property on="Test Ring" class="Ring (strict)"("Visible"=TRUE) -> ()  [unwired: 2 in, 2 out]
                n198 = property on="Test Slider" class="Slide (strict)"("Visible"=FALSE) -> ()  [unwired: 2 in, 2 out]
              }
              frame "Color Enable  **" {
                n199 = Index Array(array=w337, index=4) -> (element=w338:cluster{string[]})
                n200 = call <vilib>:"NT Read String.vi"("Name"=w340) -> ("String"=w339:string)  [unwired: 9 in, 1 out]
                n201 = Unbundle(w338) -> (w334:string[])
                n202 = Match First String(2:w334, 3:w339) -> (0:w335:i32)  [unwired: 1 out]
                n203 = property on="Test Ring" class="Ring (strict)"("Value"=w335, "Strings []"=w334) -> ()  [unwired: 2 in, 2 out]
                n204 = property on="Test Ring" class="Ring (strict)"("Visible"=TRUE) -> ()  [unwired: 2 in, 2 out]
                n205 = property on="Test Slider" class="Slide (strict)"("Visible"=FALSE) -> ()  [unwired: 2 in, 2 out]
              }
              frame Default {
                n206 = property on="Test Ring" class="Ring (strict)"("Visible"=FALSE) -> ()  [unwired: 2 in, 2 out]
                n207 = property on="Test Slider" class="Slide (strict)"("Visible"=FALSE) -> ()  [unwired: 2 in, 2 out]
              }
              frame "Brightness  **", "Color Level  **", "Compression  **", "FPS  **", "Sharpness  **" {
                n208 = call <vilib>:"NT Read Number.vi"("Name"=w346) -> ("Numeric"=w345:dbl)  [unwired: 9 in, 1 out]
                n209 = local write "Test Slider"(w345) -> ()
                n210 = property on="Test Slider" class="Slide (strict)"("Visible"=TRUE, "Scale.Maximum"=100.0 ("Scale.Range:Maximum")) -> ()  [unwired: 2 in, 2 out]
                n211 = property on="Test Ring" class="Ring (strict)"("Visible"=FALSE) -> ()  [unwired: 2 in, 2 out]
              }
            }
          }
        }
        n212 = property on="Progress" class="Clust (strict)"("Visible"=FALSE) -> ()  [unwired: 2 in, 2 out]
      }
      event "Test Name": Mouse Enter {
        # "Populate the ring with the list of tests"
        n213 = event-data() -> ()  [unwired: 1 in, 1 out]
        n214 = call <vilib>:"NT Read String Array.vi"("Name"="TestMode/TestList") -> ("String Array"=w354:string[])  [unwired: 9 in, 1 out]
        n215 = Build Array (concatenate)("Select the test to run...", w354) -> (w353:string[])
        n216 = property on="Test Name" class="Ring (strict)"("Strings []"=w353) -> ()  [unwired: 2 in, 2 out]
      }
      event "Test Name": Value Change {
        w356 = FALSE ("Visible")
        # "Tell the robot the test name to run"
        n217 = event-data() -> ("NewVal"=w360:u16)  [unwired: 1 in]
        n218 = property on="Test Name" class="Ring (strict)"() -> ("Strings []"=w361:string[])  [unwired: 2 in, 2 out]
        n219 = local write "Progress"(T6 {"Test Progress"=0, "Test Progress Text"=""} ("Progress")) -> ()
        n220 = Index Array(array=w361, index=w360) -> (element=w359:string)
        n221 = call <vilib>:"NT Write String.vi"("String"=w359, "Name"="TestMode/TestName") -> ()  [unwired: 9 in, 1 out]
        n222 = property on="Progress" class="Clust (strict)"("Visible"=TRUE) -> ()  [unwired: 2 in, 2 out]
        n223 = property on="Motor" class="Clust (strict)"("Visible"=w356) -> ()  [unwired: 2 in, 2 out]
        n224 = property on="Test Slider" class="Slide (strict)"("Visible"=w356) -> ()  [unwired: 2 in, 2 out]
        n225 = property on="On/Off" class="Bool (strict)"("Visible"=w356) -> ()  [unwired: 2 in, 2 out]
        n226 = property on="Rev/Fwd" class="Clust (strict)"("Visible"=w356) -> ()  [unwired: 2 in, 2 out]
        n227 = property on="Test Ring" class="Ring (strict)"("Visible"=w356) -> ()  [unwired: 2 in, 2 out]
      }
      event "Select Auto": Mouse Enter {
        # "Populate the combo box with the list of autonomous options"
        n228 = event-data() -> ()  [unwired: 1 in, 1 out]
        n229 = call <vilib>:"NT Read String Array.vi"("Name"="Auto List") -> ("String Array"=w363:string[])  [unwired: 9 in, 1 out]
        n230 = property on="Select Auto" class="CmbBox"("Strings[]"=w363) -> ()  [unwired: 2 in, 2 out]
      }
      event "Select Auto": Value Change {
        # "User modified the Auto Selection. Write to NT variable so robot knows."
        n231 = event-data() -> ("NewVal"=w366:string)  [unwired: 1 in]
        n232 = call <vilib>:"NT Write String.vi"("String"=w366, "Name"="Auto Selector") -> ()  [unwired: 9 in, 1 out]
      }
      event "Select Robot Start Location": Mouse Enter {
        # "Populate the combo box with the list of autonomous options"
        n233 = event-data() -> ()  [unwired: 1 in, 4 out]
        n234 = call <vilib>:"NT Read String Array.vi"("Name"="Robot Start Location List") -> ("String Array"=w369:string[])  [unwired: 9 in, 1 out]
        n235 = property on="Select Robot Start Location" class="CmbBox"("Strings[]"=w369) -> ()  [unwired: 2 in, 2 out]
      }
      event "Select Robot Start Location": Value Change {
        # "User modified the Robot Start Location Selector. Write to NT variable so robot knows."
        n236 = event-data() -> ("NewVal"=w372:string)  [unwired: 1 in]
        n237 = call <vilib>:"NT Write String.vi"("String"=w372, "Name"="Robot Start Location Selector") -> ()  [unwired: 9 in, 1 out]
      }
      event "Command Selection": Value Change {
        # "Get the params and show in table"
        n238 = event-data() -> ("NewVal"=w378:i32)  [unwired: 1 in]
        n239 = property on="Command Selection" class="MCListbox (strict)"() -> ("ItemNames"=w376:string[][])  [unwired: 2 in, 2 out]
        n240 = call <vilib>:"WPI_DashboardUpdate Command Params.vi"("NewVal"=w378, "Commands"=w376, "Param Tbl"=w377) -> ()  [unwired: 8 in, 1 out]
      }
      event "Execute Command": Value Change {
        # "Started one, Unique ID holds\nresponse"
        n241 = event-data() -> ()  [unwired: 1 in, 1 out]
        n242 = property on="Command Selection" class="MCListbox (strict)"() -> ("ItemNames"=w389:string[][])  [unwired: 2 in, 2 out]
        n243 = Index Array(array=w389, index (row)="Command Selection", index (col)=0) -> (element=w387:string)
        n244 = call <vilib>:"Invoke Commands.vi"("Command Params"="Command Params", "Function Name"=w387) -> ("Params"=w383:u8, "Started"=w382:bool)  [unwired: 7 in, 1 out]
        n245 = Array Subset(array="Command Params", length (row)=w383) -> (w384:string[][])  [unwired: 3 in]
        n246 = Select(t="Executing" ("Cmd Status"), s=w382, f="" ("Cmd Status")) -> (s? t:f=→"Cmd Status":string)
      }
      event "Command Selection": Double Click {
        n247 = event-data() -> ("Row"=w397:i32)  [unwired: 1 in]
        n248 = local read "Command Params"() -> (w396:string[][])
        n249 = property on="Command Selection" class="MCListbox (strict)"() -> ("ItemNames"=w400:string[][])  [unwired: 2 in, 2 out]
        n250 = Index Array(array=w400, index (row)=w397, index (col)=0) -> (element=w398:string)
        n251 = call <vilib>:"Invoke Commands.vi"("Command Params"=w396, "Function Name"=w398) -> ("Params"=w395:u8, "Started"=w390:bool)  [unwired: 7 in, 1 out]
        n252 = Array Subset(array=w396, length (row)=w395) -> (w394:string[][])  [unwired: 3 in]
        n253 = Select(t="Executing" ("Cmd Status"), s=w390, f="" ("Cmd Status")) -> (s? t:f=w391:string)
        n254 = local write "Cmd Status"(w391) -> ()
      }
      event "CheckList": Double Click {
        # "Shift clears all"
        # "Update symbols on the listbox"
        n255 = event-data() -> ("PlatMods.Shift"=w402:bool, "Row"=w404:i32)  [unwired: 1 in]
        n256 = case shown="True" w402 {
          tunnel: w404 -> [w408 _]
          tunnel: 1 -> [w407 _]
          frame False {
            n257 = property on="CheckList" class="LstBox (strict)"() -> ("Item Symbols"=w406:i32[])  [unwired: 2 in, 2 out]
            n258 = Replace Array Subset(array=w406, new element=w407, index=w408) -> (w405:i32[])
            n259 = property on="CheckList" class="LstBox (strict)"("Item Symbols"=w405) -> ()  [unwired: 2 in, 2 out]
          }
          frame True {
            w409 = 0 ("Top Row")
            n260 = property on="CheckList" class="LstBox (strict)"() -> ("Number of Rows"=w411:u32)  [unwired: 2 in, 2 out]
            n261 = Initialize Array(0, w411) -> (w410:i32[])
            n262 = property on="CheckList" class="LstBox (strict)"("Top Row"=w409, "Value"=w409, "Item Symbols"=w410) -> ()  [unwired: 2 in, 2 out]
          }
        }
      }
      event "CheckList": Key Down {
        # "Update symbols on the listbox\nLeft and right keys check and uncheck"
        n263 = event-data() -> ("VKey"=w415:T21)  [unwired: 1 in]
        n264 = case shown="\"Left\", \"Right\"" w415 {
          selector: w415 -> [w420 _]
          tunnel: eventvkey."Left" ("VKey") -> [w418 _]
          frame "Left", "Right" {
            n265 = Equal?(x=w418, y=w420) -> (x = y?=w419:bool)
            n266 = Select(t=0, s=w419, f=1) -> (s? t:f=w421:i32)
            n267 = property on="CheckList" class="LstBox (strict)"() -> ("Item Symbols"=w424:i32[])  [unwired: 2 in, 2 out]
            n268 = Replace Array Subset(array=w424, new element=w421, index="CheckList") -> (w423:i32[])
            n269 = property on="CheckList" class="LstBox (strict)"("Item Symbols"=w423) -> ()  [unwired: 2 in, 2 out]
          }
          frame Default {
          }
        }
      }
      event "Motor.Enable": Value Change {
        # "When the test mode otor enable helper is set, update that\ntree row item's value"
        n270 = event-data() -> ("NewVal"=w430:bool)  [unwired: 1 in]
        n271 = Unbundle("Motor") -> ("Value"=w429:dbl)  [unwired: 1 out]
        n272 = Select(t=w429, s=w430, f=0.0) -> (s? t:f=w427:dbl)
        n273 = call <vilib>:"NT Write Number.vi"("Numeric"=w427, "Name"=w426) -> ()  [unwired: 9 in, 1 out]
      }
      event "Test Slider": Value Change {
        # "When the test mode slider helper is set, update that\ntree row item's value"
        n274 = event-data() -> ("NewVal"=w433:dbl)  [unwired: 1 in]
        n275 = call <vilib>:"NT Write Number.vi"("Numeric"=w433, "Name"=w434) -> ()  [unwired: 9 in, 1 out]
      }
      event "On/Off": Value Change {
        # "When the test mode on/off helper value is set, update that\ntree row item's value"
        n276 = event-data() -> ("NewVal"=w438:bool)  [unwired: 1 in]
        n277 = Boolean To (0,1)(Boolean=w438) -> (0, 1=w437:i16)
        n278 = call <vilib>:"NT Write Number.vi"("Numeric"=w437, "Name"=w436) -> ()  [unwired: 9 in, 1 out]
      }
      event "Rev/Fwd": Value Change {
        # "When the test mode helper value for relays is set, update that\ntree row item's value"
        n279 = event-data() -> ("NewVal.Forward"=w446:bool, "NewVal.Reverse"=w445:bool)  [unwired: 1 in]
        n280 = Boolean To (0,1)(Boolean=w446) -> (0, 1=w442:i16)
        n281 = Boolean To (0,1)(Boolean=w445) -> (0, 1=w444:i16)
        n282 = Negate(x=w444) -> (-x=w443:i16)
        n283 = Add(x=w442, y=w443) -> (x+y=w441:i16)
        n284 = call <vilib>:"NT Write Number.vi"("Numeric"=w441, "Name"=w440) -> ()  [unwired: 9 in, 1 out]
      }
      event "Test Ring": Value Change {
        # "When a test mode helper value is selected from the ring,\nset the tree item's variable to the string value"
        n285 = event-data() -> ("NewVal"=w450:u16)  [unwired: 1 in]
        n286 = property on="Test Ring" class="Ring (strict)"() -> ("Strings []"=w451:string[])  [unwired: 2 in, 2 out]
        n287 = Index Array(array=w451, index=w450) -> (element=w449:string)
        n288 = call <vilib>:"NT Write String.vi"("String"=w449, "Name"=w448) -> ()  [unwired: 9 in, 1 out]
      }
      event "Rec Mode": Value Change {
        # "Update globals for recording mode and path to read log from.\nClear when logging and let NetworkTables set path for vision to\nuse."
        n289 = event-data() -> ("NewVal"=w462:enum32{"Stop", "Record", "Playback"})  [unwired: 1 in]
        n290 = global write "WPI_DashboardLogging Global.vi" "Logging Filename"(path "") -> ()
        n291 = global write "WPI_DashboardLogging Global.vi" "Recording"(w462) -> ()
        n292 = case shown="\"Playback\"" w462 {
          tunnel: w461 -> [_ w464 w473]
          tunnel: [_ _ w472] -> w459
          tunnel: [_ _ w471] -> _
          tunnel: w457 -> [_ _ w469]
          tunnel: cluster{i32, i32} {-250, 170} -> [_ _ w468]
          tunnel: [_ _ T22 {"Image Size"=TRUE, "Image Type"=TRUE, "Pixel Value"=TRUE, "ROI Information"=TRUE, "Zoom Factor"=FALSE} ("Image Information Shown:All Elements")] -> w452
          tunnel: [_ _ TRUE ("Zoom Factor")] -> w453
          tunnel: w455 -> [_ _ w465]
          frame Default {
          }
          frame "Stop", "Record" {
            # "Place Window too"
            n293 = invoke class="VI" method="FP.Close"(reference=w464) -> (reference out=w463:refnum<vi>)  [unwired: 2 in, 2 out]
            n294 = invoke class="VI" method="Abort VI"(reference=w463) -> ()  [unwired: 2 in, 3 out]
          }
          frame "Playback" {
            n295 = call "Open Playback Panel.vi"("Offset"=w468, "DB VI Ref"=w469, "Playback in"=w473) -> ("Playback out"=w470:refnum<vi>)  [unwired: 8 in]
            n296 = register-events(w470, w465) -> (reference out=w472:refnum<event-registration>, error out=w471:errorcluster)  [unwired: 2 in]
          }
        }
        n297 = property on="Camera Image Right" class="ImageControl"("Image Information Shown"=w452, "Image Information Visible"=w453) -> ()  [unwired: 2 in, 2 out]
        n298 = property on="Camera Image" class="ImageControl"("Image Information Shown"=w452, "Image Information Visible"=w453) -> ()  [unwired: 2 in, 2 out]
        n299 = call <vilib>:"WPI_DashboardNT Log FieldName Cache.vi"("Operation"=enum16{"Lookup/Add", "Index", "Clear"}."Clear") -> ()  [unwired: 8 in, 3 out]
      }
      event Panel Close {
        w475 = enum32{"Stop", "Record", "Playback"}."Stop" ("Rec Mode")
        # "Playback window has been closed, abort"
        n300 = event-data() -> ()  [unwired: 1 in, 4 out]
        n301 = local write "Rec Mode"(w475) -> ()
        n302 = global write "WPI_DashboardLogging Global.vi" "Recording"(w475) -> ()
      }
      event Panel Close {
        # "Abort playback window and ourself"
        n303 = event-data() -> ()  [unwired: 1 in, 4 out]
        n304 = invoke class="VI" method="FP.Close"(reference=w479) -> (reference out=w478:refnum<vi>)  [unwired: 2 in, 2 out]
        n305 = invoke class="VI" method="Abort VI"(reference=w478) -> (error out=w477:errorcluster)  [unwired: 2 in, 2 out]
        n306 = invoke class="VI" method="Abort VI"(error in=w477) -> ()  [unwired: 2 in, 3 out]
      }
      event User Event {
        n307 = event-data() -> ("IDs"=w486:cluster{"RPC field ID":u16, "Unique ID":u16}, "String"=w485:string)  [unwired: 1 in]
        n308 = Bundle("IDs"=w486, "String"=w485) -> (w484:T9)  [unwired: 1 in]
        n309 = call <vilib>:"Retrieve RPC Response.vi"("RPC Response"=w484) -> ("Output"=w482:string[][])  [unwired: 10 in]
        n310 = Build Array (concatenate)(w480, w482) -> (w481:string[][])
        n311 = local write "Command Params"(w481) -> ()
        n312 = local write "Cmd Status"("" ("Cmd Status")) -> ()
      }
      event "Tree": Double Click {
        n313 = event-data() -> ("PlatMods"=w492:T25, "Tag"=w489:string)  [unwired: 1 in]
        n314 = Unbundle(w492) -> ("Shift"=w491:bool)  [unwired: 4 out]
        n315 = String Subset(string=w489, length (rest)=1 ("length (rest)")) -> (substring=w488:string)  [unwired: 1 in]
        n316 = Not(x=w491) -> (.not. x?=w490:bool)
        n317 = case shown="\"/\"" w488 {
          tunnel: w489 -> [_ w495]
          tunnel: w490 -> [_ w494]
          frame Default {
          }
          frame "/" {
            n318 = call <vilib>:"NT Update Persistence.vi"("Persistence"=w494, "Name"=w495) -> ()  [unwired: 9 in, 1 out]
          }
        }
      }
    }
  }
  n319 = Index Array(array=w69) -> (element=w67:refnum<vi>)  [unwired: 1 in]
  n320 = while {
    tunnel: w67 -> [w497]
    i -> [w500]
    stop <- FALSE stop-if-true
    n321 = Wait (ms)(milliseconds to wait=u32 100) -> ()  [unwired: 1 out]
    n322 = case shown="\"Playback\"" "Rec Mode" {
      tunnel: w500 -> [_ _ w515]
      tunnel: [u32 2829099 ("Base Color") u32 11141120 ("Target Color") w504] -> w496
      frame "Stop", Default {
        # "Reset the color, extra updates don't cost much"
      }
      frame "Record" {
      }
      frame "Playback" {
        # "Playback"
        n323 = Quotient & Remainder(x=w515, y=u32 50 ("milliseconds to wait")) -> (x-y*floor(x/y)=w511:u32)  [unwired: 1 out]
        n324 = Divide(x=w511, y=u32 50 ("milliseconds to wait")) -> (x/y=w508:dbl)
        n325 = Multiply(x=6.283185307179586, y=w508) -> (x*y=w513:dbl)
        n326 = Sine(x=w513) -> (sin(x)=w512:dbl)
        n327 = Absolute Value(x=w512) -> (abs(x)=w505:dbl)
        n328 = call "Interpolate RGB Color.vi"("Proportion"=w505, "Target Color"=u32 30976, "Base Color"=u32 2829099) -> ("Result Color"=w504:u32)  [unwired: 8 in]
      }
    }
    n329 = property class="Pane"(reference=w497, "PaneColor"=w496) -> ()  [unwired: 1 in, 2 out]
  }
  n330 = local write "Dashboard Tab"(T2."Drive" ("Dashboard Tab")) -> ()
  n331 = property on="On/Off" class="Bool (strict)"("Visible"=w38) -> ()  [unwired: 2 in, 2 out]
  n332 = property on="Motor" class="Clust (strict)"("Visible"=w38) -> ()  [unwired: 2 in, 2 out]
  n333 = property on="Progress" class="Clust (strict)"("Visible"=w38) -> ()  [unwired: 2 in, 2 out]
  n334 = property on="Test Ring" class="Ring (strict)"("Visible"=w38) -> ()  [unwired: 2 in, 2 out]
  n335 = property on="Rev/Fwd" class="Clust (strict)"("Visible"=w38) -> ()  [unwired: 2 in, 2 out]
  n336 = while {
    tunnel: u16 1741 ("timeout ms (25000)") -> [w517]
    stop <- FALSE stop-if-true
    n337 = TCP Create Listener(10:w517) -> (0:w516:errorcluster, 3:w518:refnum<k5>)  [unwired: 4 in, 1 out]
    n338 = case shown="No Error" w516 {
      selector: w516 -> [w520 _]
      tunnel: w518 -> [w521 _]
      frame No Error {
        n339 = while {
          tunnel: w521 -> [w524]
          tunnel: w520 -> [w523]
          stop <- FALSE stop-if-true
          n340 = TCP Wait On Listener(8:w523, 11:w524) -> (0:w525:errorcluster, 4:w526:refnum<k5>)  [unwired: 2 in, 3 out]
          n341 = local write "TCP"(w526) -> ()
          n342 = case shown="No Error" w525 {
            frame No Error {
            }
            frame Error {
              n343 = Wait (ms)(milliseconds to wait=u32 1000) -> ()  [unwired: 1 out]
            }
          }
        }
      }
      frame Error {
        n344 = Wait (ms)(milliseconds to wait=u32 1000) -> ()  [unwired: 1 out]
      }
    }
  }
  n345 = local write "Command Selection"(u16 0 ("milliseconds to wait")) -> ()
  n346 = local write "Command Params"(string[][] [] ("Command Params")) -> ()
  n347 = global write "WPI_DashboardLogging Global.vi" "Recording"(w61) -> ()
  n348 = local write "Rec Mode"(w61) -> ()
  n349 = call <vilib>:"NT Write String.vi"("String"="Select Auto", "Name"="Auto Selector") -> ()  [unwired: 9 in, 1 out]
  n350 = call <vilib>:"NT Write String.vi"("String"="Select Robot Start Location", "Name"="Robot Start Location Selector") -> ()  [unwired: 9 in, 1 out]
